vi "valve_generic_liq_coarse.vi"(0 "PID Gains Cluster Ref":refnum<vi>, 1 "Accept Autotune":bool, 2 "Controller Toggle (Manual Mode)":bool, 3 "Valve Manual Adjust":dbl, 5 "Slide Refnum in":refnum<vi>, 7 "file (use dialog)":path, 9 "Desired Setpoint":dbl, 11 "PID gains":T2, 12 "Current Process Variable Value":dbl, 13 "autotune? (F)":bool, 14 "Reinitialize Controller":bool) -> (4 "output to valve":dbl, 6 "output to slide":dbl, 8 "tuning completed?":bool, 10 "plant parameters out":T1, 15 "PID gains out":T2)   [LabVIEW 2017]
uses:
  <vilib>/addons/control/pid/autopid.llb/PID autotuning parameters (FO).ctl
  <vilib>/addons/control/pid/NI_PID_autopid.lvlib
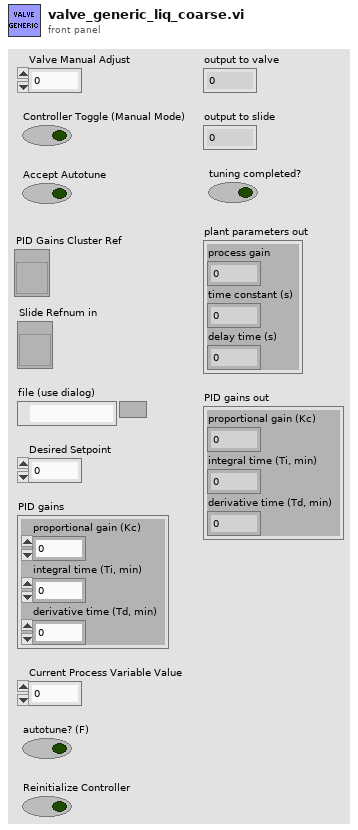
[diagram p1: front panel]
types:
  T1 = cluster{"process gain":dbl, "time constant (s)":dbl, "delay time (s)":dbl}
  T2 = cluster{"proportional gain (Kc)":dbl, "integral time (Ti, min)":dbl, "derivative time (Td, min)":dbl}
  T3 = typedef "NI_PID_autopid.lvlib/PID autotuning parameters (FO).ctl" = cluster{"type of controller":u16, "time constant factor":dbl, "step amplitude":dbl}
  T4 = enum8{"Enabled", "Disabled", "Disabled and Grayed Out"}
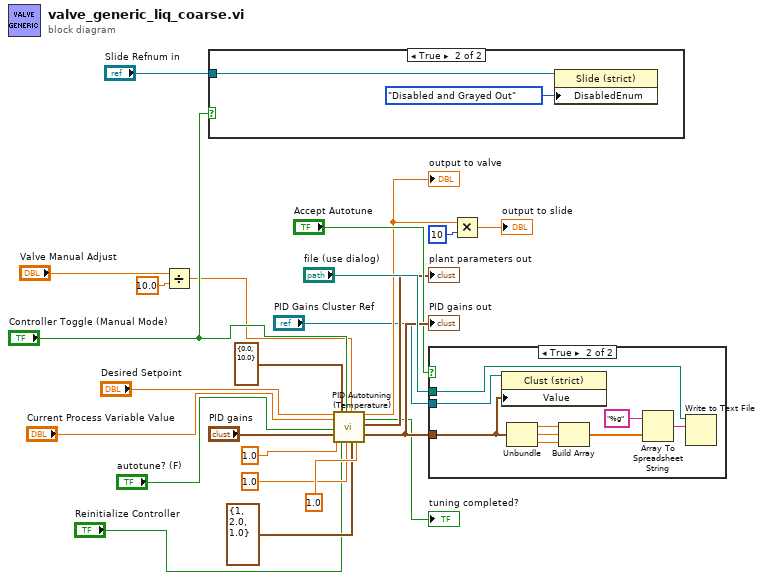
[diagram p0: block diagram]
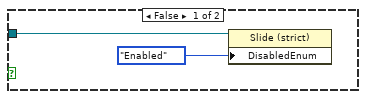
[diagram p3: hidden frame]
diagram:
  n1 = Divide(x="Valve Manual Adjust", y=10.0) -> (x/y=w12:dbl)
  n2 = case shown="True" "Controller Toggle (Manual Mode)" {
    tunnel: "Slide Refnum in" -> [w25 w28]
    frame False {
      n3 = property on="Property Node" class="Slide (strict)"(reference=w25, "DisabledEnum"=T4."Enabled" ("Disabled")) -> ()  [unwired: 1 in, 2 out]
    }
    frame True {
      n4 = property on="Property Node" class="Slide (strict)"(reference=w28, "DisabledEnum"=T4."Disabled and Grayed Out" ("Disabled")) -> ()  [unwired: 1 in, 2 out]
    }
  }
  n5 = call <vilib>:"PID Autotuning (Temperature).vi"("desired temperature"="Desired Setpoint", "measured temperature"="Current Process Variable Value", "autotune? (F)"="autotune? (F)", "PID gains in"="PID gains", "dt (s)"=1.0, "output range"=cluster{"output high":dbl, "output low":dbl} {"output high"=0.0, "output low"=10.0}, "reinitialize? (F)"="Reinitialize Controller", "auto? (T)"="Controller Toggle (Manual Mode)", "beta"=1.0, "manual control"=w12, "autotuning parameters"=T3 {"type of controller"=1, "time constant factor"=2.0, "step amplitude"=1.0}, "alpha"=1.0) -> ("output"=w9:dbl, "tuning completed?"=→"tuning completed?":bool, "plant parameters out"=→"plant parameters out":T1, "PID gains out"=w22:T2)  [unwired: 4 in]
  "PID gains out" <- w22
  "output to valve" <- w9
  n6 = case shown="True" "Accept Autotune" {
    tunnel: w22 -> [_ w37]
    tunnel: "file (use dialog)" -> [_ w30]
    tunnel: "PID Gains Cluster Ref" -> [_ w29]
    frame False {
    }
    frame True {
      n7 = property class="Clust (strict)"(reference=w29, "Value"=w37) -> ()  [unwired: 1 in, 2 out]
      n8 = Unbundle(w37) -> ("proportional gain (Kc)"=w36:dbl, "integral time (Ti, min)"=w35:dbl, "derivative time (Td, min)"=w34:dbl)
      n9 = Build Array(w36, w35, w34) -> (w33:dbl[])
      n10 = Array To Spreadsheet String(array=w33, 3:"%g" ("format string")) -> (spreadsheet string=w32:string)  [unwired: 1 in]
      n11 = Write to Text File(file (use dialog)=w30, text=w32) -> ()  [unwired: 2 in, 3 out]
    }
  }
  n12 = Multiply(x=w9, y=10) -> (x*y=→"output to slide":dbl)
